vi "TestSCAN2.vi"(8 "errin":errorcluster) -> (0 "error out":errorcluster, 2 "Tableau 2":refnum<visa-resource-name>[](array[refnum]), 3 "Tableau":string[](array[string]))   [LabVIEW 2020]
doc: "Ce VI te sniff tout les équipement VISA qu'il détect et t'en fait une liste"
uses:
  <vilib>/Instr/_visa.llb/VISA Find Search Mode.ctl
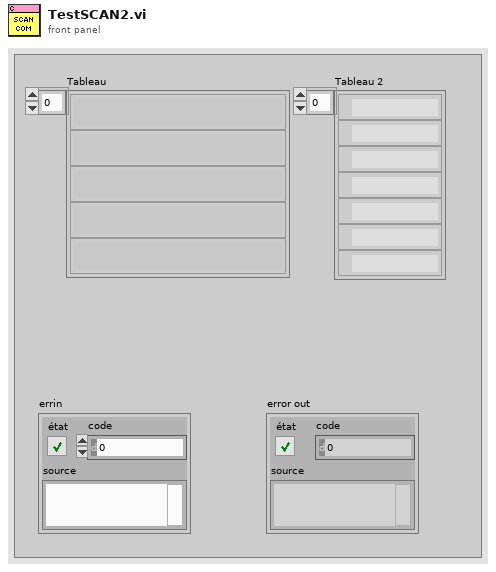
[diagram p1: front panel]
types:
  T1 = typedef "VISA Find Search Mode.ctl" = u32
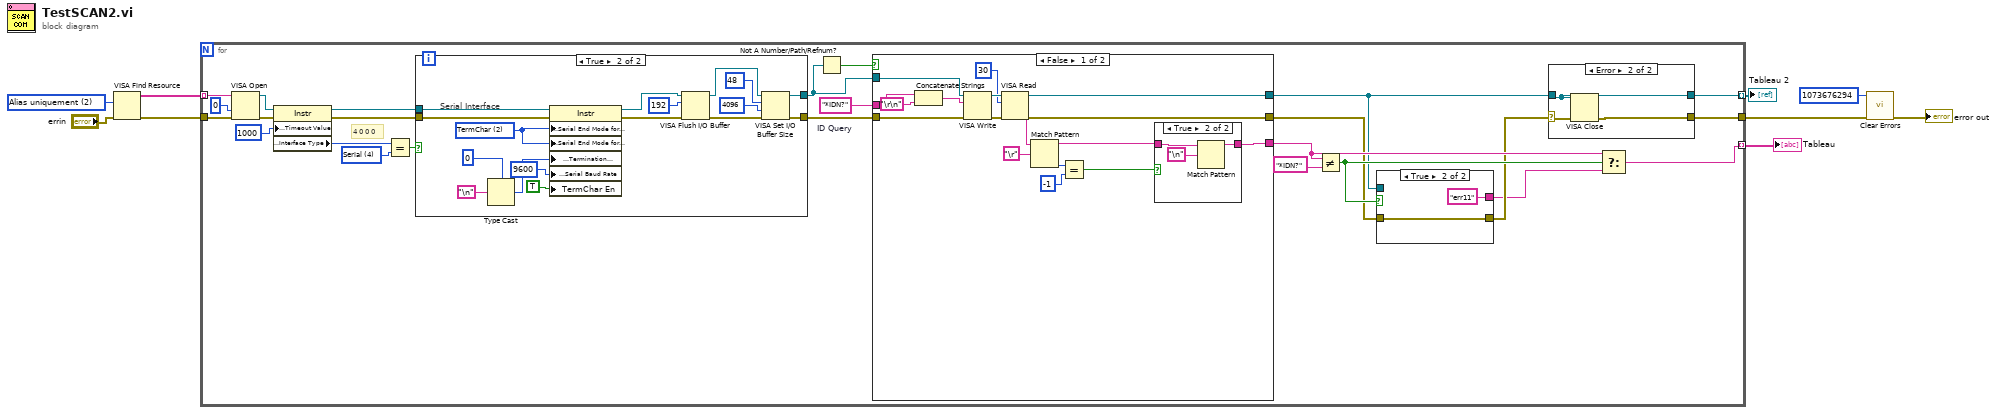
[diagram p0: block diagram]
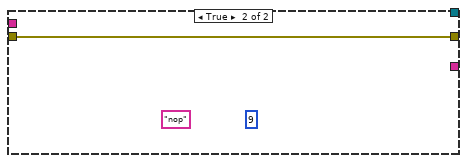
[diagram p3: hidden frame]
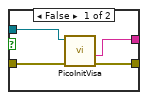
[diagram p5: hidden frame]
diagram:
  w5 = T1 2 items=["Noms canoniques uniquement"=0, "Alias uniquement"=2, "Inclure les alias correspondants"=3, "Inclure tous les alias"=4] ("Search Mode")
  n1 = VISA Find Resource(8:"errin", 10:w5) -> (0:w4:errorcluster, 3:w9:string[])  [unwired: 1 in, 1 out]
  n2 = for {
    tunnel: w9 -> [w27] mode=indexing
    tunnel: [w13] -> w8 mode=indexing
    tunnel: [w22] -> w6 mode=indexing
    tunnel: w4 -> [w26]
    tunnel: [w23] -> w3
    w24 = "*IDN?"  # ID Query
    w21 = u16 4 items=["GPIB"=1, "VXI"=2, "GPIB-VXI"=3, "Serial"=4, "PXI"=5, "TCPIP"=6, "USB"=7] ("Interface Information:Interface Type")
    # "4 0 0 0"
    n3 = VISA Open(access mode=u32 0, error in (no error)=w26, VISA resource name=w27) -> (VISA resource name=w29:refnum<visa-resource-name>, error out=w28:errorcluster)  [unwired: 2 in]
    n4 = property class="Instr"(reference=w29, error in=w28, "General Settings:Timeout Value"=u32 1000) -> (reference out=w32:refnum<visa-resource-name>, error out=w31:errorcluster, "Interface Information:Interface Type"=w12:u16)
    n5 = Equal?(x=w12, y=w21) -> (x = y?=w10:bool)
    n6 = case shown="True" w10 {
      tunnel: [w57 w72] -> w33
      tunnel: [w58 w69] -> w11
      tunnel: w32 -> [w57 w74]
      tunnel: w31 -> [w58 w75]
      frame False {
        # "EDIT: Remove interfaces not supported by your instrument."
        # "GPIB, TCP/IP, and USB Interface"
      }
      frame True {
        w62 = u16 2 items=["None", "LastBit", "TermChar"] ("Serial Settings:Serial End Mode for Reads")
        # "Serial Interface"
        n7 = Type Cast(type=u8 0, x="\n" ("Line Feed Constant")) -> (*(type *) &x=w61:u8)
        n8 = property class="Instr"(reference=w74, error in=w75, "Serial Settings:Serial End Mode for Reads"=w62, "Serial Settings:Serial End Mode for Writes"=w62, "Message Based Settings:Termination Character"=w61, "Serial Settings:Serial Baud Rate"=u32 9600 ("Serial Settings:Baud Rate"), "TermChar En"=TRUE ("Message Based Settings:Termination Character Enable")) -> (reference out=w68:refnum<visa-resource-name>, error out=w71:errorcluster)
        n9 = VISA Flush I/O Buffer(VISA resource name=w68, mask (16)=u16 192, error in (no error)=w71) -> (VISA resource name out=w73:refnum<visa-resource-name>, error out=w70:errorcluster)
        n10 = VISA Set I/O Buffer Size(VISA resource name=w73, mask (16)=u16 48, size (4096)=u32 4096 ("size (0)"), error in (no error)=w70) -> (VISA resource name out=w72:refnum<visa-resource-name>, error out=w69:errorcluster)
      }
    }
    n11 = Not A Number/Path/Refnum?(number/path/refnum=w33) -> (NaN/Path/Refnum?=w25:bool)
    n12 = case shown="False" w25 {
      tunnel: [w37 _] -> w15
      tunnel: [w39 w56] -> w17
      tunnel: [w45 _] -> w19
      tunnel: w33 -> [w38 _]
      tunnel: w24 -> [w44 _]
      tunnel: w11 -> [w42 w56]
      frame False {
        n13 = Concatenate Strings(w44, "\r\n") -> (w48:string)
        n14 = VISA Write(VISA resource name=w38, write buffer=w48, error in (no error)=w42) -> (VISA resource name out=w51:refnum<visa-resource-name>, error out=w50:errorcluster)  [unwired: 1 out]
        n15 = VISA Read(VISA resource name=w51, byte count=u32 30 ("nombre d'octets"), error in (no error)=w50) -> (VISA resource name out=w37:refnum<visa-resource-name>, read buffer=w41:string, error out=w39:errorcluster)  [unwired: 1 out]
        n16 = Match Pattern(string=w41, regular expression="\r") -> (before substring=w36:string, offset past match=w40:i32)  [unwired: 1 in, 2 out]
        n17 = Equal?(x=w40, y=-1) -> (x = y?=w35:bool)
        n18 = case shown="True" w35 {
          tunnel: w36 -> [w52 w54]
          tunnel: [w52 w53] -> w45
          frame False {
          }
          frame True {
            n19 = Match Pattern(string=w54, regular expression="\n") -> (before substring=w53:string)  [unwired: 1 in, 3 out]
          }
        }
      }
      frame True {
        (unwired) 9 ("offset past match")
        (unwired) "nop" ("read buffer")
      }
    }
    n20 = Not Equal?(x=w19, y="*IDN?") -> (x != y?=w18:bool)
    n21 = case shown="True" w18 {
      tunnel: w17 -> [w79 w81]
      tunnel: [w78 w81] -> w16
      tunnel: w15 -> [w77 _]
      tunnel: [w76 "err11" ("data out")] -> w14
      frame False {
        n22 = call "PicoInitVisa.vi"("errin"=w79, "visain"=w77) -> ("sortie d'erreur"=w78:errorcluster, "buffer de lecture 2"=w76:string)  [unwired: 6 in, 2 out]
      }
      frame True {
      }
    }
    n23 = case shown="Error" w16 {
      selector: w16 -> [w82 w86]
      tunnel: w15 -> [w83 w84]
      tunnel: [w83 w84] -> w22
      tunnel: [w82 w85] -> w23
      frame No Error {
      }
      frame Error {
        n24 = VISA Close(VISA resource name=w84, error in (no error)=w86) -> (error out=w85:errorcluster)
      }
    }
    n25 = Select(t=w19, s=w18, f=w14) -> (s? t:f=w13:string)
  }
  "Tableau" <- w8
  "Tableau 2" <- w6
  n26 = call <vilib>:"Clear Errors.vi"("error in (no error)"=w3, "specific error code to clear (0: all)"=1073676294) -> ("error out"=→"error out":errorcluster)  [unwired: 4 in, 1 out]
